vi "JLINKARM TIF Select.vi"(8 "error in (no error)":errorcluster, 11 "Interface":i32) -> (0 "error out":errorcluster, 3 "function return":i32)   [LabVIEW 2020, in "JLinkARM.lvlib"]
doc: "JLINKARMDLL_API int JLINKARM_TIF_Select (int Interface);"
uses:
  Lib/JLinkARM.lvlib
  JLinkARM.dll
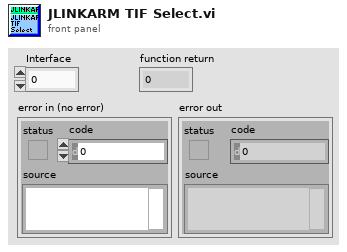
[diagram p1: front panel]
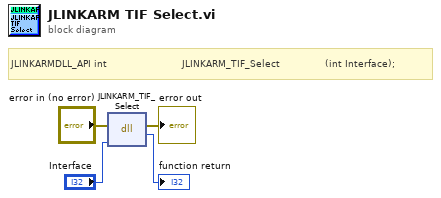
[diagram p0: block diagram]
diagram:
  # "JLINKARMDLL_API int                         JLINKARM_TIF_Select               (int Interface);"
  n1 = dll-call lib="C:/Users/anybody/Desktop/JLinkARM.*" fn="JLINKARM_TIF_Select"(error in="error in (no error)", "Interface"="Interface") -> (error out=→"error out":errorcluster, →"function return":i32)  [unwired: 3 in, 1 out]
